vi "CleanUp.vi"(0 "object in":refnum<class "AFG3022B.lvclass">, 5 "error in (no error)":errorcluster) -> (14 "object out":refnum<class "AFG3022B.lvclass">, 19 "error out":errorcluster)   [LabVIEW 2019, in "AFG3022B.lvclass"]
uses:
  AFG3022B.lvclass
  AFG3022B.lvclass/AFG3022B.ctl
  Tektronix AFG 3000 Series/Tektronix AFG 3000 Series.lvlib
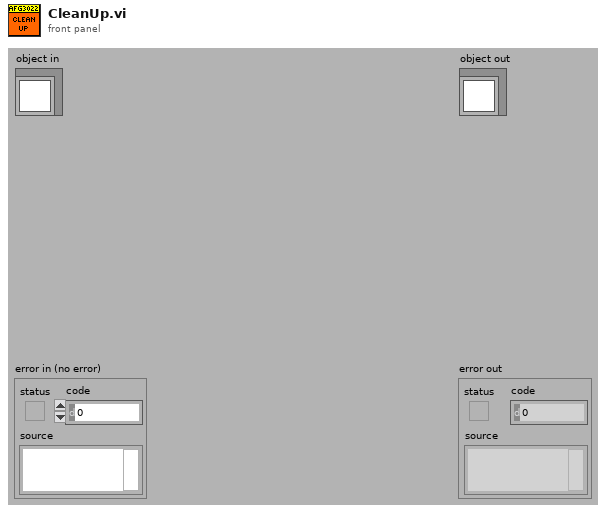
[diagram p1: front panel]
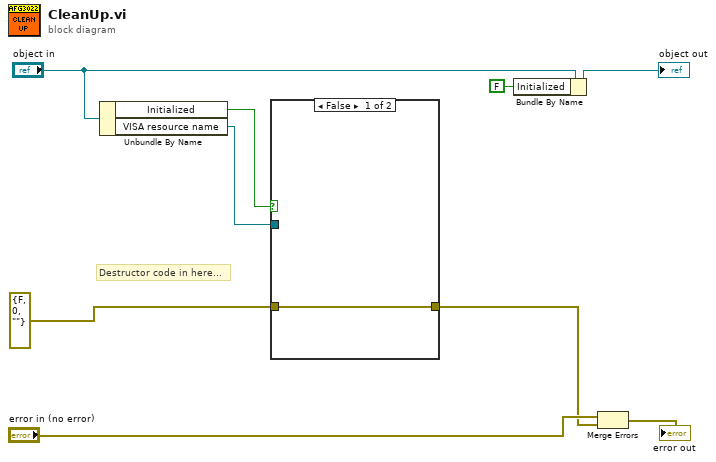
[diagram p0: block diagram]
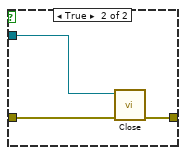
[diagram p2: hidden frame]
diagram:
  # "Destructor code in here..."
  n1 = Unbundle By Name("object in") -> ("Initialized"=w6:bool, "VISA resource name"=w5:refnum<visa-resource-name>)
  n2 = case shown="False" w6 {
    tunnel: errorcluster {"status"=FALSE, "code"=0, "source"=""} ("error in (no error)") -> [w10 w12]
    tunnel: w5 -> [_ w13]
    tunnel: [w10 w11] -> w3
    frame False {
    }
    frame True {
      n3 = call "Close.vi"("error in (no error)"=w12, "VISA resource name"=w13) -> ("error out"=w11:errorcluster)  [unwired: 9 in]
    }
  }
  n4 = Bundle By Name(cluster="object in", "Initialized"=FALSE) -> (→"object out":refnum<class "AFG3022B.lvclass">)
  n5 = Merge Errors("error in (no error)", w3) -> (→"error out":errorcluster)
